vi "Thorlabs Module.vi"(7 "Actions":T3(ring)=enum."Generate Scan Pattern", 8 "error in":errorcluster, 9 "Objective":u16(ring)=1 items=["5X LKM05", "10X LKM10", "20X LKM20", "10X LSM02"], 10 "ROI Parameters":T1={"ROI (mm)"={"X (mm)"=1.0, "Y (mm)"=1.0}, "Shift (mm)"={"Xshift (mm)"=0.0, "Yshift (mm)"=0.0}}, 11 "Scan Parameters":T2={"# Scan"={"#Ascan"=400, "#Bscan"=400}, "# Rpt"={"#ARpt"=1, "#BRpt"=1}, "Aline Rate"=2, "# Extra"={"# ARpt_extra"=5, "#Brtn_extra"=60}} {"Aline Rate" items=["76 KHz", "146 KHz", "76 KHz", "28 KHz", "10 KHz"]}) -> (0 "error out":errorcluster, 2 "Data Out":sgl[][](array[numeric]), 3 "Raw Data Out":u16[][](array[numeric]))   [LabVIEW 2017]
uses:
  Hardware/Thorlabs OCT/user.lib/SpectralRadar.llb/Processing Flag Selection.ctl
  Hardware/Thorlabs OCT/user.lib/SpectralRadar.llb/Probe Parameter Int Selection.ctl
  Hardware/Thorlabs OCT/user.lib/SpectralRadar.llb/Scan Pattern.lvclass
  Hardware/Thorlabs OCT/user.lib/SpectralRadar.llb/set Spectrum Output.vi
  Hardware/Thorlabs OCT/user.lib/SpectralRadar.llb/set Scan Output.vi
  Hardware/Thorlabs OCT/user.lib/SpectralRadar.llb/Data.lvclass
  Hardware/Thorlabs OCT/user.lib/SpectralRadar.llb/Raw Data.lvclass
  Hardware/Thorlabs OCT/user.lib/SpectralRadar.llb/Processing.lvclass
  Hardware/Thorlabs OCT/user.lib/SpectralRadar.llb/Probe.lvclass
  Hardware/Thorlabs OCT/user.lib/SpectralRadar.llb/OCT Device.lvclass
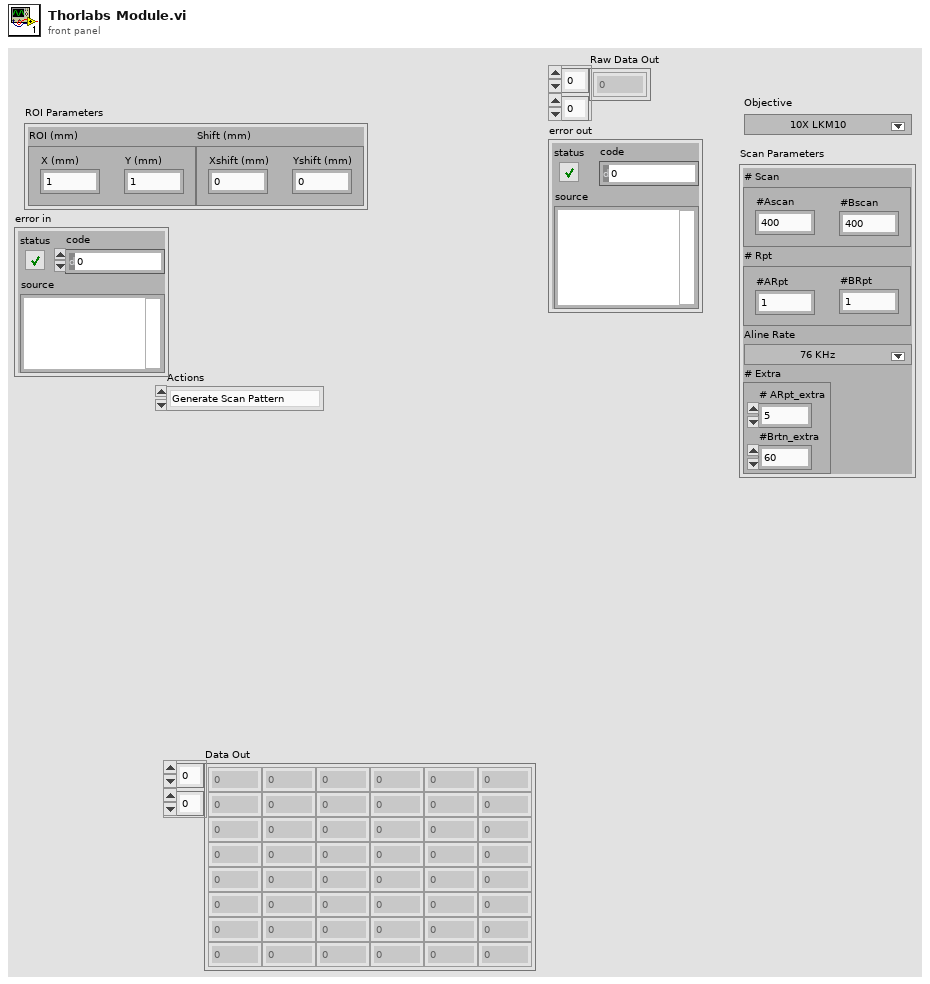
[diagram p1: front panel]
types:
  T1 = cluster{"ROI (mm)":cluster{"X (mm)":dbl, "Y (mm)":dbl}, "Shift (mm)":cluster{"Xshift (mm)":sgl, "Yshift (mm)":sgl}}
  T2 = cluster{"# Scan":cluster{"#Ascan":i32, "#Bscan":i32}, "# Rpt":cluster{"#ARpt":i32, "#BRpt":i32}, "Aline Rate":u16, "# Extra":cluster{"# ARpt_extra":i32, "#Brtn_extra":i32}}
  T3 = enum16{"Init", "Configure", "Configure Data", "Generate Scan Pattern", "Start Acquire Raw", "Start Acquire Data", "Acquire RAW", "Acquire Data", "Stop Acquire", "Uninit"}
  T4 = typedef "Processing.lvclass/Processing Flag Selection.ctl" = enum16{"Use Offset Errors", "Remove DC Spectrum", "Remove Advanced DC Spectrum", "Use Apodization", "Use Scan For Apodization", "Filter Undersampled Signals", "Use Dispersion Compensation", "Use Dechirp", "Use Extended Adjust", "Full Range Output", "Filter DC", "Autocorrelation Compensation", "DEFR", "Only Windowing", "Remove Fixed Pattern"}
  T5 = enum16{"FreeRunning", "TrigBoard_ExternalStart", "External_AScan"}
  T6 = typedef "Probe.lvclass/Probe Parameter Int Selection.ctl" = enum16{"Apodization Cycles", "Oversampling", "White Balance Auto", "Oversampling Slow Axis"}
  T7 = enum16{"Asynchronous Continuous", "Asynchronous Finite", "Synchronous"}
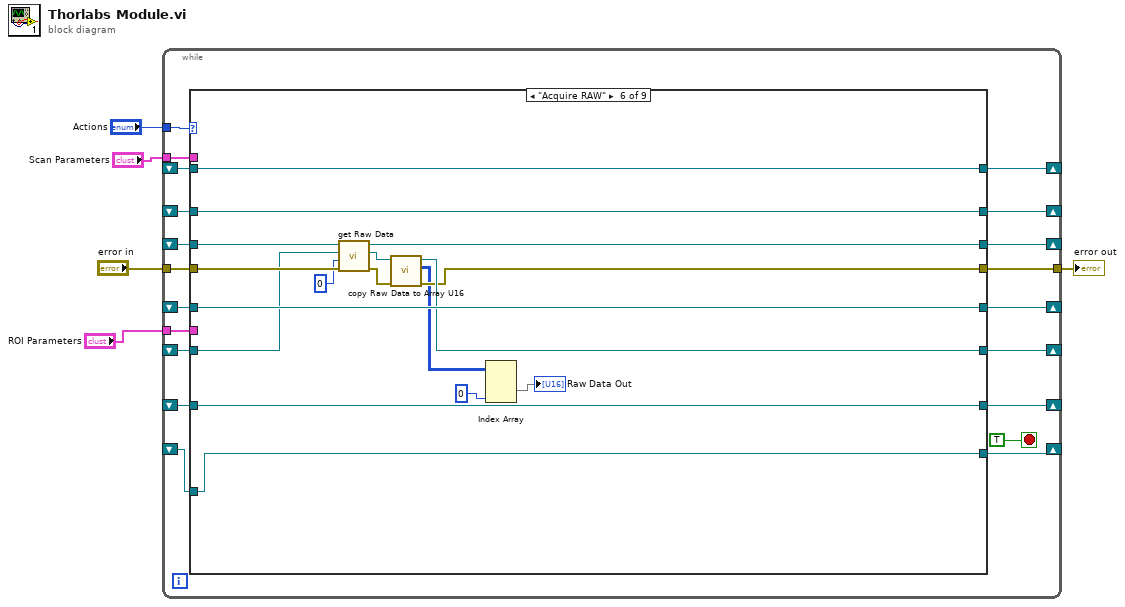
[diagram p0: block diagram]
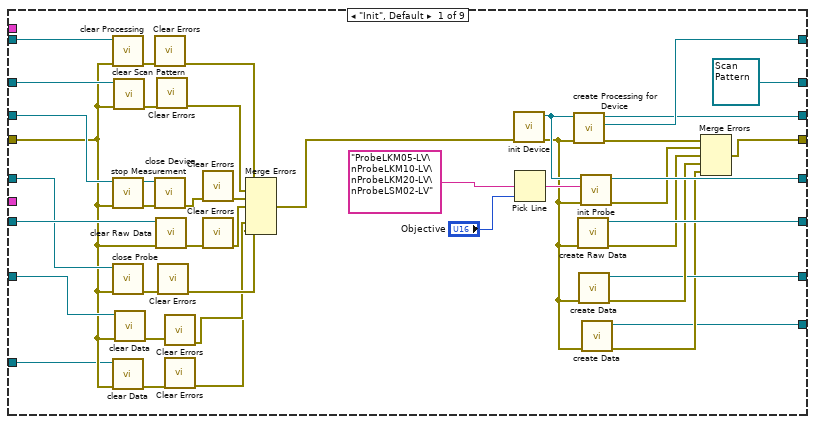
[diagram p2: hidden frame]
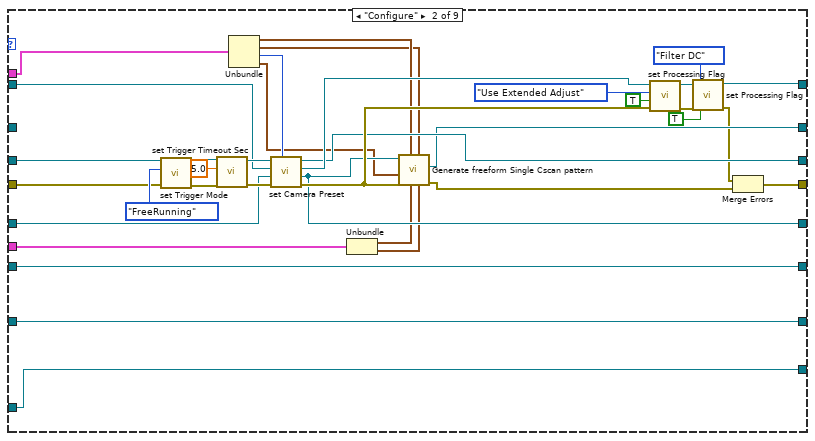
[diagram p3: hidden frame]
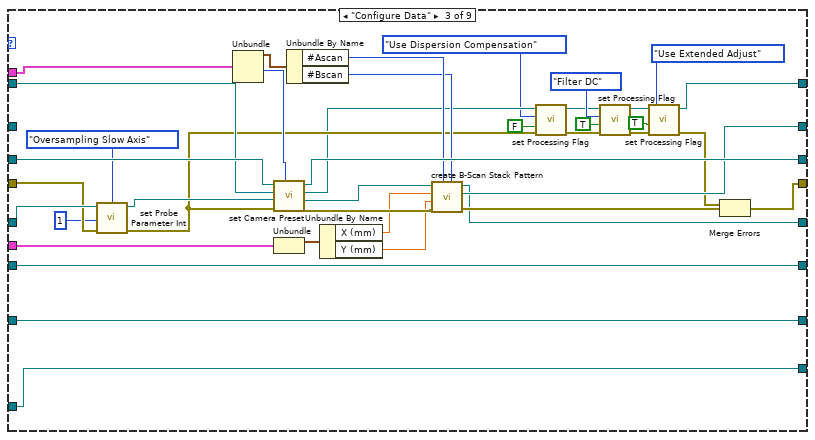
[diagram p4: hidden frame]
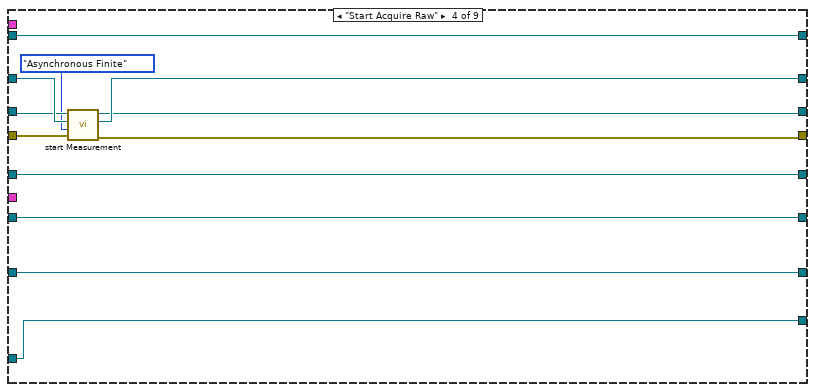
[diagram p5: hidden frame]
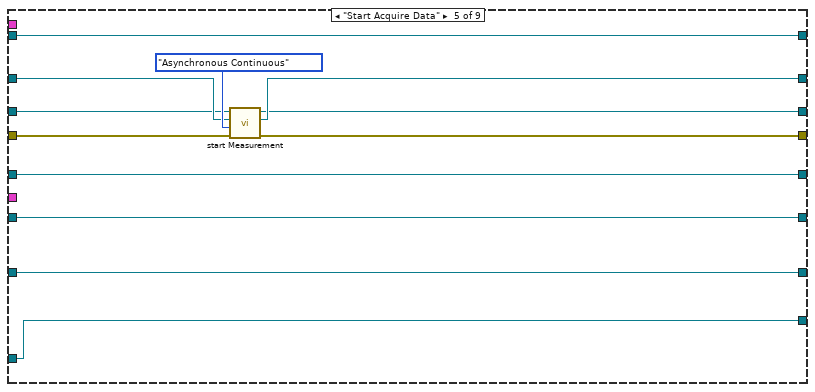
[diagram p6: hidden frame]
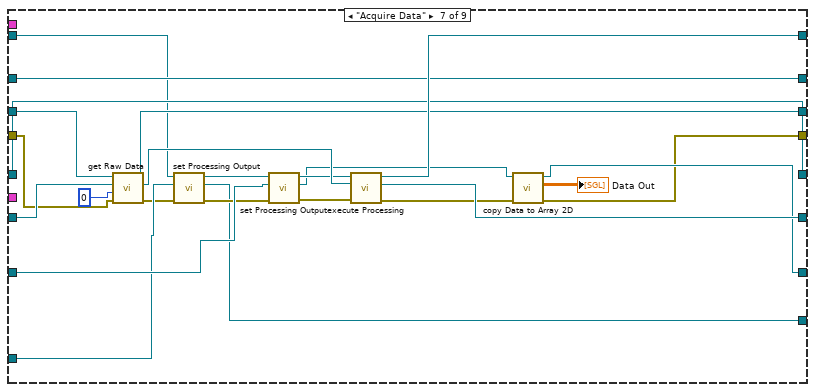
[diagram p7: hidden frame]
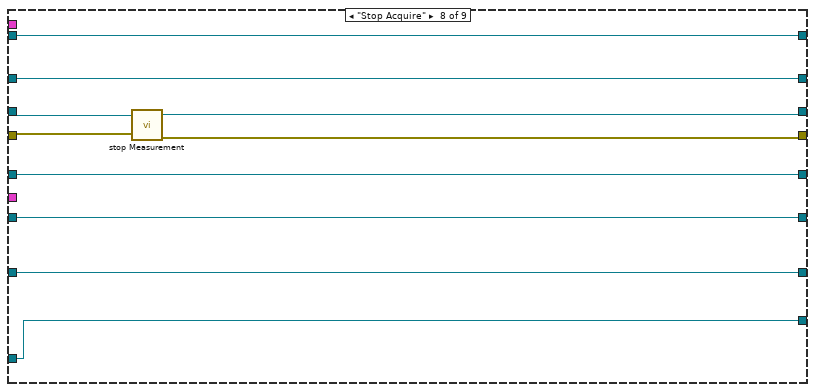
[diagram p8: hidden frame]
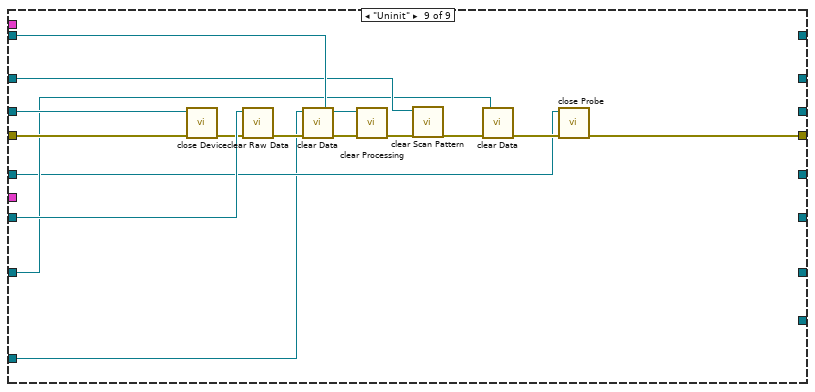
[diagram p9: hidden frame]
diagram:
  n1 = while {
    tunnel: "Actions" -> [w25]
    shift-right: [w23] -> _
    shift-left: _ -> [w19]
    shift-right: [w20] -> _
    shift-left: _ -> [w18]
    shift-right: [w17] -> _
    shift-left: _ -> [w16]
    shift-right: [w15] -> _
    shift-left: _ -> [w14]
    shift-right: [w13] -> _
    shift-left: _ -> [w12]
    tunnel: "error in" -> [w21]
    tunnel: [w22] -> w4
    shift-right: [w11] -> _
    shift-left: _ -> [w10]
    shift-right: [w9] -> _
    shift-left: _ -> [w8]
    tunnel: "Scan Parameters" -> [w7]
    tunnel: "ROI Parameters" -> [w6]
    stop <- TRUE stop-if-true
    n2 = case shown="\"Acquire RAW\"" w25 {
      tunnel: [w55 w91 w140 w151 w162 w179 w201 w216 _] -> w23
      tunnel: [w61 w103 w127 w155 w166 w174 w186 w218 w224] -> w22
      tunnel: w21 -> [w30 w81 w137 w156 w167 w183 w200 w219 w228]
      tunnel: [w63 w92 w122 w149 w160 w184 w203 w213 _] -> w20
      tunnel: w19 -> [w52 w80 w141 w152 w163 w181 w208 w217 w232]
      tunnel: w18 -> [w49 w75 w139 w149 w160 w184 w203 w213 w223]
      tunnel: [w57 w71 w106 w150 w161 w185 w205 w214 _] -> w17
      tunnel: w16 -> [w47 w82 w134 w150 w161 w185 w197 w214 w231]
      tunnel: [w64 w94 w125 w148 w159 w175 w202 w212 _] -> w15
      tunnel: w14 -> [w50 w94 w125 w148 w159 w180 w209 w212 w234]
      tunnel: [refnum<class "Scan Pattern.lvclass"> refnum ("Scan Pattern") w90 w126 w153 w164 w178 w204 w215 _] -> w13
      tunnel: w12 -> [w48 _ _ w154 w165 w178 w204 w215 w229]
      tunnel: [w42 w79 w124 w146 w158 w170 w189 w211 _] -> w11
      tunnel: w10 -> [w40 w79 w124 w146 w158 w170 w199 w211 w227]
      tunnel: [w31 w78 w123 w145 w157 w169 w188 w210 _] -> w9
      tunnel: w8 -> [w27 w78 w123 w145 w157 w169 w198 w210 w220]
      tunnel: w7 -> [_ w77 w121 _ _ _ _ _ _]
      tunnel: w6 -> [_ w76 w120 _ _ _ _ _ _]
      frame "Init", Default {
        n3 = call "clear Processing.vi"("error in (no error)"=w30, "Processing"=w47) -> ("error out"=w46:errorcluster)  [unwired: 5 in]
        n4 = call "stop Measurement.vi"("error in (no error)"=w30, "OCTDevice"=w52) -> ("error out"=w54:errorcluster, "OCTDevice"=w53:refnum<class "OCT Device.lvclass">)  [unwired: 4 in]
        n5 = call "close Probe.vi"("error in (no error)"=w30, "GalvoControl"=w49) -> ("error out"=w45:errorcluster)  [unwired: 5 in]
        n6 = call "clear Data.vi"("error in (no error)"=w30, "Data"=w27) -> ("error out"=w29:errorcluster)  [unwired: 5 in]
        n7 = call "clear Scan Pattern.vi"("error in (no error)"=w30, "Scan Pattern in"=w48) -> ("error out"=w44:errorcluster)  [unwired: 5 in]
        n8 = call "clear Data.vi"("error in (no error)"=w30, "Data"=w40) -> ("error out"=w41:errorcluster)  [unwired: 5 in]
        n9 = call <vilib>:"Clear Errors.vi"("error in (no error)"=w46) -> ("error out"=w39:errorcluster)  [unwired: 5 in, 1 out]
        n10 = call "close Device.vi"("error in (no error)"=w54, "OCTDevice"=w53) -> ("error out"=w66:errorcluster)  [unwired: 5 in]
        n11 = call "clear Raw Data.vi"("error in (no error)"=w30, "Raw Data"=w50) -> ("error out"=w65:errorcluster)  [unwired: 5 in]
        n12 = call <vilib>:"Clear Errors.vi"("error in (no error)"=w44) -> ("error out"=w38:errorcluster)  [unwired: 5 in, 1 out]
        n13 = call <vilib>:"Clear Errors.vi"("error in (no error)"=w45) -> ("error out"=w35:errorcluster)  [unwired: 5 in, 1 out]
        n14 = call <vilib>:"Clear Errors.vi"("error in (no error)"=w41) -> ("error out"=w34:errorcluster)  [unwired: 5 in, 1 out]
        n15 = call <vilib>:"Clear Errors.vi"("error in (no error)"=w29) -> ("error out"=w28:errorcluster)  [unwired: 5 in, 1 out]
        n16 = call <vilib>:"Clear Errors.vi"("error in (no error)"=w66) -> ("error out"=w37:errorcluster)  [unwired: 5 in, 1 out]
        n17 = call <vilib>:"Clear Errors.vi"("error in (no error)"=w65) -> ("error out"=w36:errorcluster)  [unwired: 5 in, 1 out]
        n18 = Merge Errors(w39, w38, w37, w36, w35, w34, w28) -> (w32:errorcluster)
        n19 = call "init Device.vi"("error in (no error)"=w32) -> ("error out"=w26:errorcluster, "OCTDevice"=w58:refnum<class "OCT Device.lvclass">)  [unwired: 5 in]
        n20 = Pick Line(multi-line string="ProbeLKM05-LV\nProbeLKM10-LV\nProbeLKM20-LV\nProbeLSM02-LV" ("string (\"\")"), line index="Objective") -> (output string=w62:string)  [unwired: 1 in]
        n21 = call "create Processing for Device.vi"("error in (no error)"=w26, "OCTDevice"=w58) -> ("error out"=w56:errorcluster, "Processing"=w57:refnum<class "Processing.lvclass">, "OCTDevice"=w55:refnum<class "OCT Device.lvclass">)  [unwired: 3 in]
        n22 = call "create Raw Data.vi"("error in (no error)"=w26) -> ("error out"=w59:errorcluster, "Raw Data"=w64:refnum<class "Raw Data.lvclass">)  [unwired: 5 in]
        n23 = call "create Data.vi"("error in (no error)"=w26) -> ("error out"=w43:errorcluster, "Data"=w42:refnum<class "Data.lvclass">)  [unwired: 5 in]
        n24 = call "init Probe.vi"("error in (no error)"=w26, "Probe"=w62, "OCT Device"=w58) -> ("error out"=w60:errorcluster, "GalvoControl"=w63:refnum<class "Probe.lvclass">)  [unwired: 3 in]
        n25 = call "create Data.vi"("error in (no error)"=w26) -> ("error out"=w33:errorcluster, "Data"=w31:refnum<class "Data.lvclass">)  [unwired: 5 in]
        n26 = Merge Errors(w56, w60, w59, w43, w33) -> (w61:errorcluster)
      }
      frame "Configure" {
        n27 = call "set Trigger Mode.vi"("error in (no error)"=w81, "Trigger Type"=T5."FreeRunning", "OCTDevice in"=w80) -> ("error out"=w102:errorcluster, "OCTDevice out"=w104:refnum<class "OCT Device.lvclass">)  [unwired: 3 in]
        n28 = call "set Trigger Timeout Sec.vi"("error in (no error)"=w102, "Trigger Timeout"=5.0, "OCTDevice in"=w104) -> ("error out"=w96:errorcluster, "OCTDevice out"=w95:refnum<class "OCT Device.lvclass">)  [unwired: 3 in]
        n29 = Unbundle(w77) -> ("# Scan"=w87:cluster{"#Ascan":i32, "#Bscan":i32}, "# Rpt"=w86:cluster{"#ARpt":i32, "#BRpt":i32}, "Aline Rate"=w88:u16, "# Extra"=w83:cluster{"# ARpt_extra":i32, "#Brtn_extra":i32})
        n30 = call "set Camera Preset.vi"("Numeric"=w88, "error in (no error)"=w96, "Probe"=w75, "Processing"=w82, "OCTDevice"=w95) -> ("error out"=w93:errorcluster, "Probe 2"=w92:refnum<class "Probe.lvclass">, "Processing"=w97:refnum<class "Processing.lvclass">, "OCTDevice out"=w91:refnum<class "OCT Device.lvclass">)  [unwired: 1 in]
        n31 = Unbundle(w76) -> ("ROI (mm)"=w85:cluster{"X (mm)":dbl, "Y (mm)":dbl}, "Shift (mm)"=w84:cluster{"Xshift (mm)":sgl, "Yshift (mm)":sgl})
        n32 = call "Generate freeform Single Cscan pattern.vi"("Shift (mm)"=w84, "# Rpt"=w86, "ROI (mm)"=w85, "# Scan"=w87, "error in (no error)"=w93, "# Extra"=w83, "Probe"=w92) -> ("error out"=w89:errorcluster, "Scan Pattern"=w90:refnum<class "Scan Pattern.lvclass">)  [unwired: 1 in, 2 out]
        n33 = call "set Processing Flag.vi"("error in (no error)"=w93, "Flag"=TRUE, "Processing Flag Selection"=Processing_Flag_Selection."Use Extended Adjust", "Processing"=w97) -> ("error out"=w74:errorcluster, "Processing"=w72:refnum<class "Processing.lvclass">)  [unwired: 2 in]
        n34 = call "set Processing Flag.vi"("error in (no error)"=w74, "Flag"=TRUE, "Processing Flag Selection"=Processing_Flag_Selection."Filter DC", "Processing"=w72) -> ("error out"=w73:errorcluster, "Processing"=w71:refnum<class "Processing.lvclass">)  [unwired: 2 in]
        n35 = Merge Errors(w73, w89) -> (w103:errorcluster)
      }
      frame "Configure Data" {
        n36 = call "set Probe Parameter Int.vi"("error in (no error)"=w137, "Value"=1, "Probe Parameter Int"=Probe_Parameter_Int_Selection."Oversampling Slow Axis", "GalvoControl"=w139) -> ("error out"=w119:errorcluster, "GalvoControl"=w138:refnum<class "Probe.lvclass">)  [unwired: 2 in]
        n37 = Unbundle(w121) -> ("# Scan"=w131:cluster{"#Ascan":i32, "#Bscan":i32}, "Aline Rate"=w144:u16)  [unwired: 2 out]
        n38 = call "set Camera Preset.vi"("Numeric"=w144, "error in (no error)"=w119, "Probe"=w138, "Processing"=w134, "OCTDevice"=w141) -> ("error out"=w133:errorcluster, "Probe 2"=w132:refnum<class "Probe.lvclass">, "Processing"=w113:refnum<class "Processing.lvclass">, "OCTDevice out"=w140:refnum<class "OCT Device.lvclass">)  [unwired: 1 in]
        n39 = Unbundle(w120) -> ("ROI (mm)"=w142:cluster{"X (mm)":dbl, "Y (mm)":dbl})  [unwired: 1 out]
        n40 = Unbundle By Name(w131) -> ("#Ascan"=w130:i32, "#Bscan"=w129:i32)
        n41 = Unbundle By Name(w142) -> ("X (mm)"=w118:dbl, "Y (mm)"=w117:dbl)
        n42 = call "create B-Scan Stack Pattern.vi"("Size Y"=w129, "Size X"=w130, "error in (no error)"=w133, "Range Y"=w117, "Range X"=w118, "Probe"=w132) -> ("error out"=w128:errorcluster, "Scan Pattern"=w126:refnum<class "Scan Pattern.lvclass">, "Probe"=w122:refnum<class "Probe.lvclass">)  [unwired: 1 in]
        n43 = call "set Processing Flag.vi"("error in (no error)"=w119, "Flag"=FALSE, "Processing Flag Selection"=Processing_Flag_Selection."Use Dispersion Compensation", "Processing"=w113) -> ("error out"=w114:errorcluster, "Processing"=w112:refnum<class "Processing.lvclass">)  [unwired: 2 in]
        n44 = call "set Processing Flag.vi"("error in (no error)"=w114, "Flag"=TRUE, "Processing Flag Selection"=Processing_Flag_Selection."Filter DC", "Processing"=w112) -> ("error out"=w143:errorcluster, "Processing"=w107:refnum<class "Processing.lvclass">)  [unwired: 2 in]
        n45 = call "set Processing Flag.vi"("error in (no error)"=w143, "Flag"=TRUE, "Processing Flag Selection"=Processing_Flag_Selection."Use Extended Adjust", "Processing"=w107) -> ("error out"=w109:errorcluster, "Processing"=w106:refnum<class "Processing.lvclass">)  [unwired: 2 in]
        n46 = Merge Errors(w109, w128) -> (w127:errorcluster)
      }
      frame "Start Acquire Raw" {
        n47 = call "start Measurement.vi"("error in (no error)"=w156, "Acquisition Type"=T7."Asynchronous Finite", "Scan Pattern"=w154, "OCTDevice"=w152) -> ("error out"=w155:errorcluster, "Scan Pattern"=w153:refnum<class "Scan Pattern.lvclass">, "OCTDevice"=w151:refnum<class "OCT Device.lvclass">)  [unwired: 1 in]
      }
      frame "Start Acquire Data" {
        n48 = call "start Measurement.vi"("error in (no error)"=w167, "Acquisition Type"=T7."Asynchronous Continuous", "Scan Pattern"=w165, "OCTDevice"=w163) -> ("error out"=w166:errorcluster, "Scan Pattern"=w164:refnum<class "Scan Pattern.lvclass">, "OCTDevice"=w162:refnum<class "OCT Device.lvclass">)  [unwired: 1 in]
      }
      frame "Acquire RAW" {
        n49 = call "get Raw Data.vi"("error in (no error)"=w183, "Camera Index"=0, "RawData in"=w180, "OCTDevice in"=w181) -> ("error out"=w177:errorcluster, "RawData out"=w176:refnum<class "Raw Data.lvclass">, "OCTDevice out"=w179:refnum<class "OCT Device.lvclass">)  [unwired: 1 in]
        n50 = call "copy Raw Data to Array U16.vi"("error in (no error)"=w177, "Data in"=w176) -> ("error out"=w174:errorcluster, "Data Content"=w172:u16[][][], "Data out"=w175:refnum<class "Raw Data.lvclass">)  [unwired: 3 in]
        n51 = Index Array(array=w172, index (dim 2)=0 ("index (page)")) -> (element=→"Raw Data Out":u16[][])  [unwired: 2 in]
      }
      frame "Acquire Data" {
        n52 = call "get Raw Data.vi"("error in (no error)"=w200, "Camera Index"=0, "RawData in"=w209, "OCTDevice in"=w208) -> ("error out"=w196:errorcluster, "RawData out"=w206:refnum<class "Raw Data.lvclass">, "OCTDevice out"=w201:refnum<class "OCT Device.lvclass">)  [unwired: 1 in]
        n53 = call-poly "set Processing Output.vi"("error in (no error)"=w196, "Data"=w198, "Processing"=w197) -> ("error out"=w195:errorcluster, "Data"=w188:refnum<class "Data.lvclass">, "Processing"=w193:refnum<class "Processing.lvclass">)  [unwired: 2 in]
        n54 = call-poly "set Processing Output.vi"("error in (no error)"=w195, "Data"=w199, "Processing"=w193) -> ("error out"=w207:errorcluster, "Data"=w191:refnum<class "Data.lvclass">, "Processing"=w192:refnum<class "Processing.lvclass">)  [unwired: 2 in]
        n55 = call "execute Processing.vi"("error in (no error)"=w207, "Raw Data"=w206, "Processing"=w192) -> ("error out"=w187:errorcluster, "Raw Data"=w202:refnum<class "Raw Data.lvclass">, "Processing"=w205:refnum<class "Processing.lvclass">)  [unwired: 2 in]
        n56 = call "copy Data to Array 2D.vi"("error in (no error)"=w187, "Data in"=w191) -> ("error out"=w186:errorcluster, "Data Content"=→"Data Out":sgl[][], "Data out"=w189:refnum<class "Data.lvclass">)  [unwired: 3 in]
      }
      frame "Stop Acquire" {
        n57 = call "stop Measurement.vi"("error in (no error)"=w219, "OCTDevice"=w217) -> ("error out"=w218:errorcluster, "OCTDevice"=w216:refnum<class "OCT Device.lvclass">)  [unwired: 4 in]
      }
      frame "Uninit" {
        n58 = call "close Device.vi"("error in (no error)"=w228, "OCTDevice"=w232) -> ("error out"=w233:errorcluster)  [unwired: 5 in]
        n59 = call "clear Raw Data.vi"("error in (no error)"=w233, "Raw Data"=w234) -> ("error out"=w222:errorcluster)  [unwired: 5 in]
        n60 = call "clear Data.vi"("error in (no error)"=w222, "Data"=w220) -> ("error out"=w221:errorcluster)  [unwired: 5 in]
        n61 = call "clear Processing.vi"("error in (no error)"=w221, "Processing"=w231) -> ("error out"=w230:errorcluster)  [unwired: 5 in]
        n62 = call "clear Scan Pattern.vi"("error in (no error)"=w230, "Scan Pattern in"=w229) -> ("error out"=w226:errorcluster)  [unwired: 5 in]
        n63 = call "clear Data.vi"("error in (no error)"=w226, "Data"=w227) -> ("error out"=w225:errorcluster)  [unwired: 5 in]
        n64 = call "close Probe.vi"("error in (no error)"=w225, "GalvoControl"=w223) -> ("error out"=w224:errorcluster)  [unwired: 5 in]
      }
    }
  }
  "error out" <- w4
